vi "CalibrationWrite.vi"(0 "handle":u64, 1 "CalArray":i32[](array[numeric]), 3 "error in (no error)":errorcluster caption="错误输入（无错误）") -> (7 "handle out":u64, 8 "function return":i32, 10 "error out":errorcluster caption="错误输出")   [LabVIEW 2018]
doc: "Write Calibration Config Array from the device's EEPROM.\nWARMING: You should Read Calibration Config Array and save the data before use this VI to ensure that the data can be recovered!!!!!!!!!!!"
panel:
  # "Carefully use this VI !!!!!!!!!!!!!!!!!\nWARMING: You should Read Calibration Config Array and save the data \nbefore use this VI to ensure that the data can be recovered !!!!!!!!!!!"
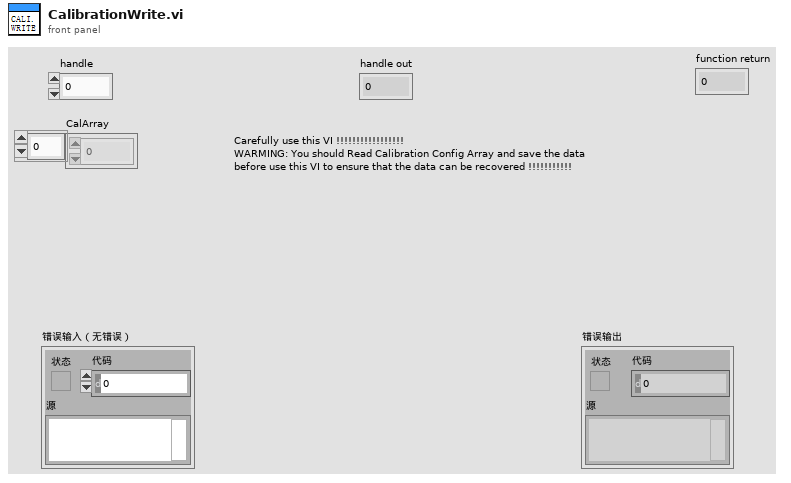
[diagram p1: front panel]
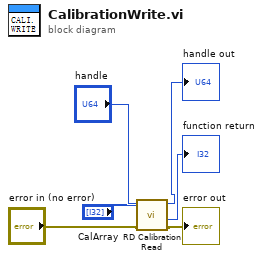
[diagram p0: block diagram]
diagram:
  n1 = call "RD Calibration Read.vi"("error in (no error)"="error in (no error)", 10:"CalArray", "handle"="handle") -> ("error out"=→"error out":errorcluster, "function return"=→"function return":i32, "handle out"=→"handle out":u64)  [unwired: 5 in, 1 out]
